vi "Read_Image.vi"(7 "PreProcessing_Options":T2={"DS_Name"="delete", "Input_Dims"={"C"=3, "H"=224, "W"=224}, "Center Crop Size"=0, "Interpolation Type"=1, "Multi-Stage_DownSample?"=FALSE, "Dataset_Stats"={"means"={"R"=0.5385, "G"=0.5348, "B"=0.551}, "stds"={"R"=0.3673, "G"=0.3673, "B"=0.3505}}} {"Dataset_Stats"."stds"."R" format="%#_3g"; "Dataset_Stats"."stds"."G" format="%#_3g"; "Dataset_Stats"."stds"."B" format="%#_3g"; "Dataset_Stats"."means"."R" format="%#_3g"; "Dataset_Stats"."means"."G" format="%#_3g"; "Dataset_Stats"."means"."B" format="%#_3g"; "Interpolation Type" items=["Zero Order", "Bi-Linear", "Quadratic", "Cubic Spline"]}, 8 "error in":errorcluster, 10 "IMAQ Name":string="train_orig", 11 "Img Path":path) -> (0 "error out":errorcluster, 2 "Imaq Image Out":T1, 3 "Image Out":sgl[][][](array[numeric]), 5 "dT_Img_Read":dbl=0.005897299968637526 format="%#_6p")   [LabVIEW 2024]
uses:
  <vilib>/Ngene/DeepLTK Anomaly Detection Addon/DeepLTK_Anomaly_Detection_Addon/API/Controls/NNPC_PreProcessing_Options.ctl
  <vilib>/Ngene/Deep Learning Toolkit/Toolkit/NN_Data/API/NN_Dims(C,H,W).ctl
  <vilib>/Ngene/DeepLTK Anomaly Detection Addon/DeepLTK_Anomaly_Detection_Addon/API/Controls/NNPC_DS_Stats.ctl
  <vilib>/Ngene/DeepLTK Anomaly Detection Addon/DeepLTK_Anomaly_Detection_Addon/API/Controls/Image_Stats_RGB.ctl
  <vilib>/vision/Image Controls.llb/IMAQ Image.ctl
  <vilib>/Ngene/Deep Learning Toolkit/Toolkit/Deep_Learning_Toolkit_by_Ngene.lvlib
  <vilib>/Ngene/DeepLTK Anomaly Detection Addon/DeepLTK_Anomaly_Detection_Addon/DeepLTK_Anomaly_Detection_Addon.lvlib
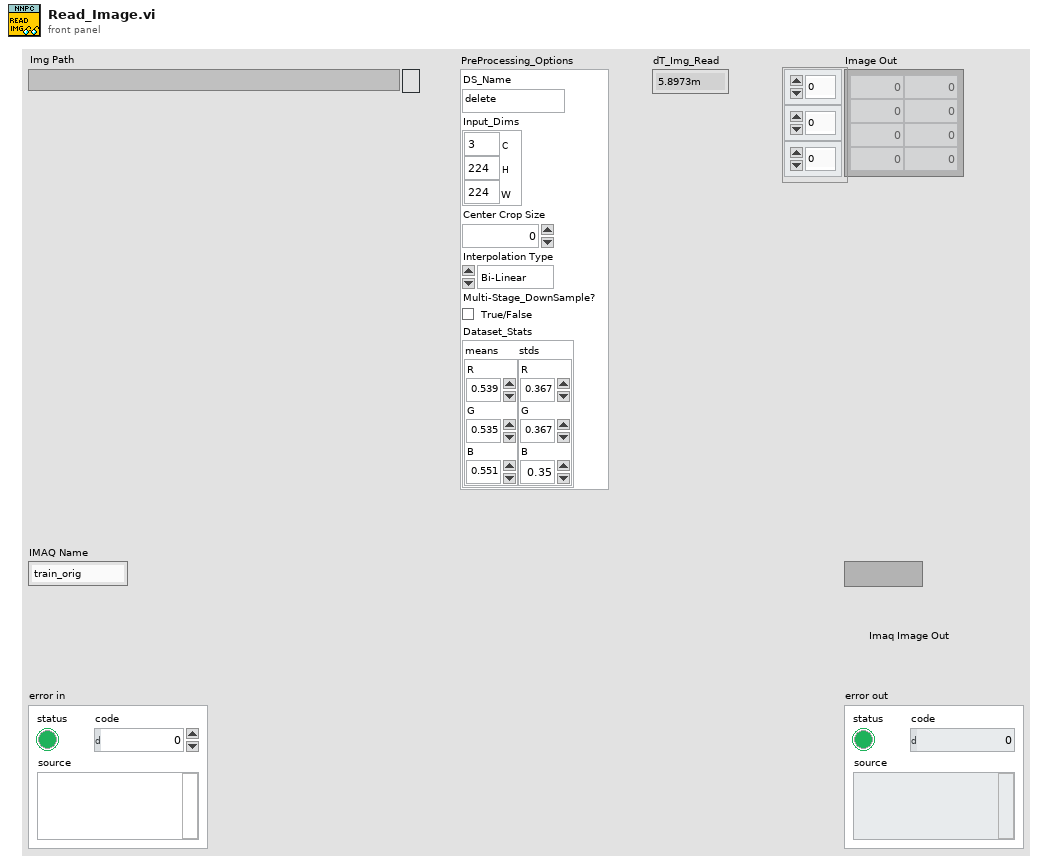
[diagram p1: front panel]
types:
  T1 = typedef "IMAQ Image.ctl" = refnum<image>
  T2 = typedef "DeepLTK_Anomaly_Detection_Addon.lvlib/NNPC_PreProcessing_Options.ctl" = cluster{"DS_Name":string, "Input_Dims":T3, "Center Crop Size":i32, "Interpolation Type":u32, "Multi-Stage_DownSample?":bool, "Dataset_Stats":T4}
  T3 = typedef "Deep_Learning_Toolkit_by_Ngene.lvlib/NN_Dims(C,H,W).ctl" = cluster{"C":i32, "H":i32, "W":i32}
  T4 = typedef "DeepLTK_Anomaly_Detection_Addon.lvlib/NNPC_DS_Stats.ctl" = cluster{"means":T5, "stds":T5}
  T5 = typedef "DeepLTK_Anomaly_Detection_Addon.lvlib/Image_Stats_RGB.ctl" = cluster{"R":sgl, "G":sgl, "B":sgl}
  T6 = typedef "Image Type" = u32
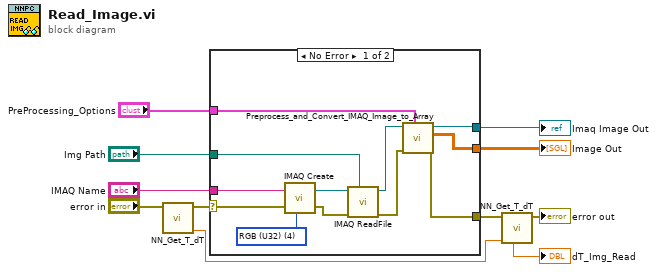
[diagram p0: block diagram]
diagram:
  n1 = call <vilib>:"NN_Get_T_dT.vi"("error in (no error)"="error in") -> ("T_out"=w4:dbl, "error out"=w7:errorcluster)  [unwired: 6 in, 1 out]
  n2 = case shown="No Error" w7 {
    selector: w7 -> [w20 w24]
    tunnel: "Img Path" -> [w22 _]
    tunnel: [w14 _] -> w9
    tunnel: [w21 w24] -> w8
    tunnel: "IMAQ Name" -> [w16 _]
    tunnel: [w13 _] -> w2
    tunnel: "PreProcessing_Options" -> [w12 _]
    frame No Error {
      w17 = T6 4 items=["Grayscale (U8)", "Grayscale (I16)", "Grayscale (SGL)", "Complex (CSG)", "RGB (U32)", "HSL (U32)", "RGB (U64)", "Grayscale (U16)"] ("Image Type")
      n3 = call "IMAQ Create"("Image Name"=w16, "Image Type"=w17, "error in (no error)"=w20) -> ("New Image"=w23:T1, "error out"=w15:errorcluster)  [unwired: 2 in]
      n4 = call "IMAQ ReadFile"("File Path"=w22, "error in (no error)"=w15, "Image"=w23) -> ("error out"=w19:errorcluster, "Image Out"=w18:T1)  [unwired: 4 in, 3 out]
      n5 = call "Preprocess_and_Convert_IMAQ_Image_to_Array.vi"("PreProcessing_Options"=w12, "error in (no error)"=w19, "Imaq Image In"=w18) -> ("error out"=w21:errorcluster, "Norm_Img_Out"=w14:sgl[][][], "Imaq Image Out"=w13:T1)  [unwired: 5 in, 1 out]
    }
    frame Error {
    }
  }
  "Image Out" <- w9
  "Imaq Image Out" <- w2
  n6 = call <vilib>:"NN_Get_T_dT.vi"("T_in"=w4, "error in (no error)"=w8) -> ("error out"=→"error out":errorcluster, "dT"=→"dT_Img_Read":dbl)  [unwired: 5 in, 1 out]
